vi "GotoWaypoint.vi"(3 "SupressIn":dbl, 7 "InhibitIn":bool, 8 "CurrentSteerAngle":dbl, 9 "WhatAroundMe? Clean":cluster{"T":dbl, "Range":dbl, "Bearing":dbl}[](array[cluster]), 10 "WhereAmI? Clean":T3, 11 "MDF In":T1) -> (0 "SupressOut":dbl, 1 "MDF Out":T1, 2 "ActCommand":dbl[](array[numeric]), 4 "InhibitOut":bool, 5 "Vel":dbl, 6 "SteerAngle":dbl)   [LabVIEW 2010]
doc: "This subVI contains the Forebrain Goto Waypoint behaviors. Its inputs are the outputs of thewhat and where SENSE processes, theMission efinition Filet, a suppression value from another co-brahvior and an inhibit signal to turn the behavior off. The outputs are a 90 element steering array and a suppression value to diminish the output of co-behaviors.\n\nIt is designed to work with a 90 element behavior arbiter."
uses:
  4-High Neurons/MDFArray.ctl
  4-High Neurons/MissionDefinitionFile.ctl
  <vilib>/Analysis/1siggen.llb/Ramp Pattern by Samples.vi
  <vilib>/gmath/statdist.llb/Normal PDF.vi
  <vilib>/gmath/NI_Gmath.lvlib
  <vilib>/Analysis/NI_AALBase.lvlib
panel:
  out "loop index":i32
  in  "HowAmI? Clean":cluster{"T":dbl, "Battery":dbl, "Temp":dbl}
  # "This VI contains the go to waypoint behavior  at the Forebrain level"
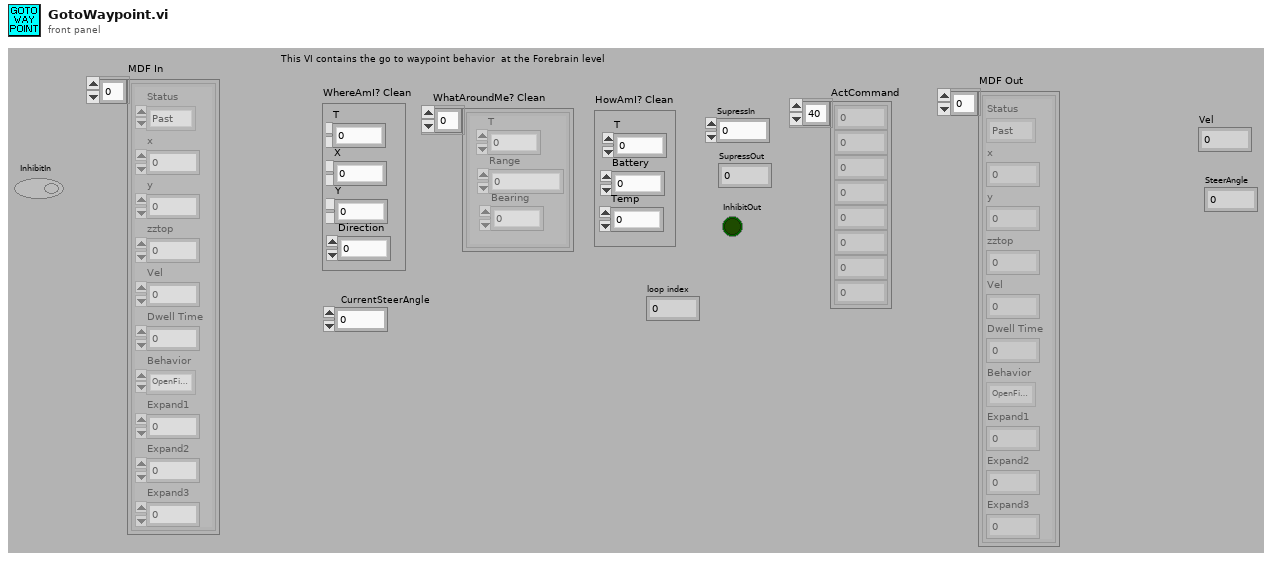
[diagram p1: front panel]
types:
  T1 = typedef "MDFArray.ctl" = T2[]
  T2 = typedef "MissionDefinitionFile.ctl" = cluster{"Status":enum16{"Past", "Current", "Future"}, "x":dbl, "y":dbl, "zztop":dbl, "Vel":dbl, "Dwell Time":dbl, "Behavior":enum16{"OpenFieldTransit", "WallFollow", "LaneFollow", "ManualMode"}, "Expand1":dbl, "Expand2":dbl, "Expand3":dbl}
  T3 = cluster{"T":dbl, "X":dbl, "Y":dbl, "Direction":dbl}
  T4 = cluster{"VelCom":dbl, "BehCom":enum16{"OpenFieldTransit", "WallFollow", "LaneFollow", "ManualMode"}}
  T5 = enum16{"OpenFieldTransit", "WallFollow", "LaneFollow", "ManualMode"}
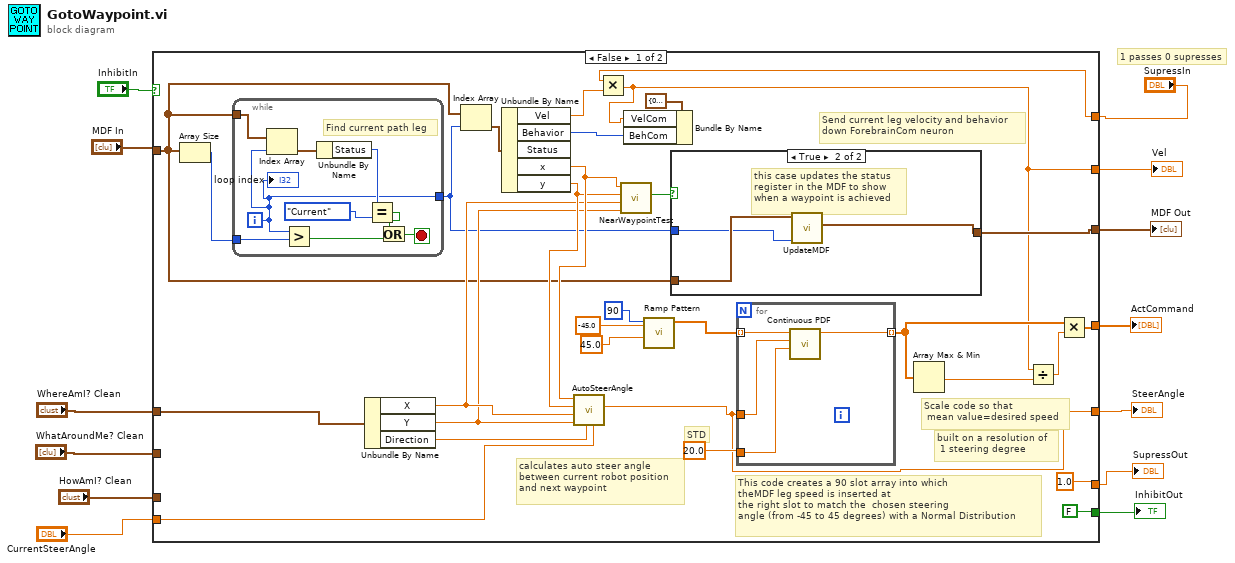
[diagram p0: block diagram]
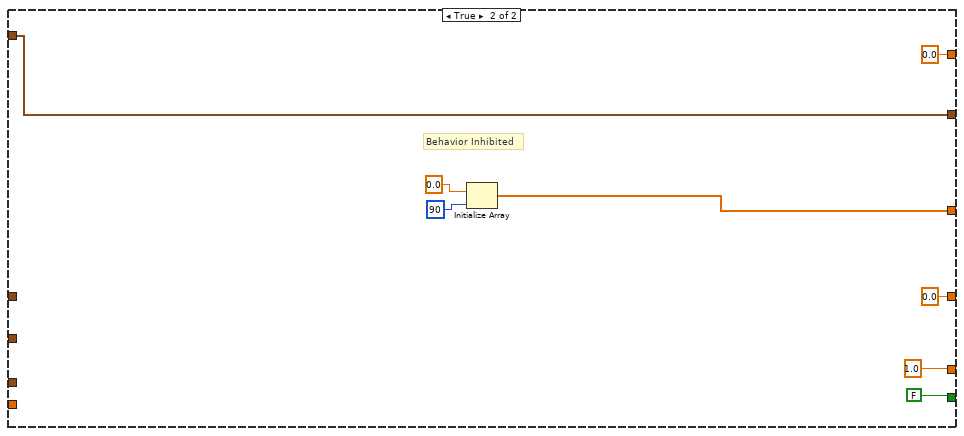
[diagram p3: hidden frame]
diagram:
  # "1 passes 0 supresses"
  n1 = case shown="False" "InhibitIn" {
    tunnel: "WhatAroundMe? Clean" -> [_ _]
    tunnel: "WhereAmI? Clean" -> [w40 _]
    tunnel: "HowAmI? Clean" -> [_ _]
    tunnel: "SupressIn" -> [w15 _]
    tunnel: [w28 w66] -> w6
    tunnel: [1.0 ("SupressOut") 1.0 ("SupressOut")] -> w8
    tunnel: [FALSE ("InhibitOut") FALSE ("InhibitOut")] -> w7
    tunnel: "MDF In" -> [w21 w63]
    tunnel: [w20 w63] -> w4
    tunnel: [w14 0.0 ("Vel")] -> w3
    tunnel: [w17 0.0 ("SteerAngle")] -> w2
    tunnel: "CurrentSteerAngle" -> [w16 _]
    frame False {
      # "calculates auto steer angle\nbetween current robot position\nand next waypoint"
      # "built on a resolution of\n 1 steering degree"
      # "Scale code so that\n mean value=desired speed"
      # "STD"
      # "This code creates a 90 slot array into which\ntheMDF leg speed is inserted at\nthe right slot to match the  chosen steering\nangle (from -45 to 45 degrees) with a Normal Distribution"
      # "Send current leg velocity and behavior\ndown ForebrainCom neuron"
      n2 = Array Size(array=w21) -> (size(s)=w41:i32)
      n3 = while {
        tunnel: w41 -> [w60]
        tunnel: w21 -> [w57]
        tunnel: [w52] -> w19
        i -> [w52]
        stop <- w59 stop-if-true
        # "Find current path leg"
        n4 = Index Array "Index Array"(array=w57, index=w52) -> (element=w54:T2)
        n5 = Greater?(x=w52, y=w60) -> (0:w58:bool)
        n6 = Unbundle By Name(w54) -> ("Status"=w55:enum16{"Past", "Current", "Future"})
        n7 = Equal?(x=w55, y=enum16{"Past", "Current", "Future"}."Current") -> (x = y?=w56:bool)
        n8 = Or(x=w56, y=w58) -> (x .or. y?=w59:bool)
        "loop index" <- w52
      }
      n9 = Unbundle By Name(w40) -> ("X"=w24:dbl, "Y"=w23:dbl, "Direction"=w27:dbl)
      n10 = Index Array "Index Array"(array=w21, index=w19) -> (element=w39:T2)
      n11 = Unbundle By Name(w39) -> ("Vel"=w18:dbl, "Behavior"=w37:T5, "x"=w26:dbl, "y"=w25:dbl)  [unwired: 1 out]
      n12 = call "AutoSteerAngle.vi"("CurrentSteerAngle"=w16, "CurrentDirection"=w27, "Ycurrent"=w23, "Xcurrent"=w24, "Ywaypoint"=w25, "Xwaypoint"=w26) -> ("NewSteerAngle"=w17:dbl)  [unwired: 5 in]
      n13 = Multiply(x=w15, y=w18) -> (x*y=w14:dbl)
      n14 = call "NearWaypointTest.vi"("Yrobot"=w23, "Xrobot"=w24, "Ywaypoint"=w25, "Xwaypoiny"=w26) -> ("AtWaypoint"=w22:bool)  [unwired: 7 in]
      n15 = Bundle By Name(cluster=T4 {"VelCom"=0.0, "BehCom"=enum."OpenFieldTransit"} ("ForebrainCom"), "VelCom"=w14, "BehCom"=w37) -> ()  [unwired: 1 out]
      n16 = call-poly <vilib>:"Ramp Pattern.vi"("start"=45.0, "end"=-45.0 ("end (Normal)"), "samples"=90) -> ("Ramp Pattern"=w31:dbl[])  [unwired: 7 in, 1 out]
      n17 = case shown="True" w22 {
        tunnel: w21 -> [w44 w47]
        tunnel: [w44 w45] -> w20
        tunnel: w19 -> [_ w46]
        frame False {
          # "robot not near waypoint\npass MDF through unaltered"
        }
        frame True {
          # "this case updates the status\nregister in the MDF to show \nwhen a waypoint is achieved"
          n18 = call "UpdateMDF.vi"("Index"=w46, "MDF_In"=w47) -> ("MDF_Out"=w45:T1)  [unwired: 9 in]
        }
      }
      n19 = for {
        tunnel: w31 -> [w51] mode=indexing
        tunnel: 20.0 ("std (Normal)") -> [w50]
        tunnel: [w49] -> w35 mode=indexing
        tunnel: w17 -> [w48]
        n20 = call-poly <vilib>:"Continuous PDF.vi"("std"=w50, "mean"=w48, "x"=w51) -> ("pdf(x)"=w49:dbl)  [unwired: 7 in, 1 out]
      }
      n21 = Array Max & Min(array=w35) -> (max value=w33:dbl)  [unwired: 3 out]
      n22 = Divide(x=w14, y=w33) -> (x/y=w34:dbl)
      n23 = Multiply(x=w35, y=w34) -> (x*y=w28:dbl[])
    }
    frame True {
      # "Behavior Inhibited"
      n24 = Initialize Array "Initialize Array"(0.0 ("element"), 90 ("dimension size")) -> (w66:dbl[])
    }
  }
  "ActCommand" <- w6
  "SupressOut" <- w8
  "InhibitOut" <- w7
  "MDF Out" <- w4
  "Vel" <- w3
  "SteerAngle" <- w2
